vi "SimpleDevice.vi"(8 "error in (no error)":errorcluster, 11 "Name":string) -> (0 "error out":errorcluster, 3 "SimpleDevice":refnum<class "SimpleDevice.lvclass">)   [LabVIEW 2021, in "SimpleDevice.lvlib" / "SimpleDevice.lvclass"]
uses:
  SimpleDevice.lvclass
  SimpleDevice.lvclass/SimpleDevice.ctl
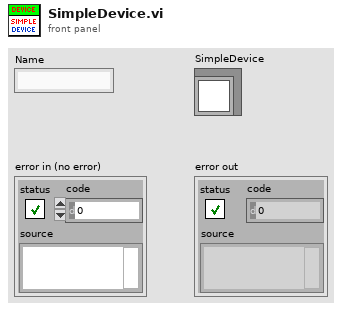
[diagram p1: front panel]
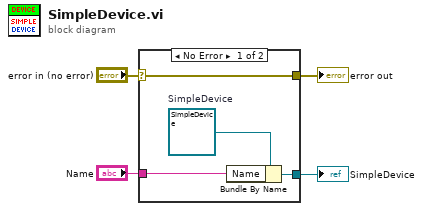
[diagram p0: block diagram]
diagram:
  n1 = case shown="No Error" "error in (no error)" {
    selector: "error in (no error)" -> [w8 w9]
    tunnel: [w8 w9] -> w3
    tunnel: [w5 _] -> w2
    tunnel: "Name" -> [w6 _]
    frame No Error {
      w7 = refnum<class "SimpleDevice.lvclass"> refnum  # SimpleDevice
      n2 = Bundle By Name(cluster=w7, "Name"=w6) -> (w5:refnum<class "SimpleDevice.lvclass">)
    }
    frame Error {
    }
  }
  "error out" <- w3
  "SimpleDevice" <- w2
